vi "Populate_Do.vi"(8 "error in (no error)":errorcluster, 9 "Value":string, 10 "Lower case name":string, 11 "Build Named Build Specification in":refnum<class "Build Named Build Specification.lvclass">) -> (0 "error out":errorcluster, 1 "Success?":bool, 3 "Build Named Build Specification out":refnum<class "Build Named Build Specification.lvclass">)   [LabVIEW 2020, in "ProjectBuilder.lvlib" / "Build Named Build Specification.lvclass"]
uses:
  Build Named Build Specification.lvclass
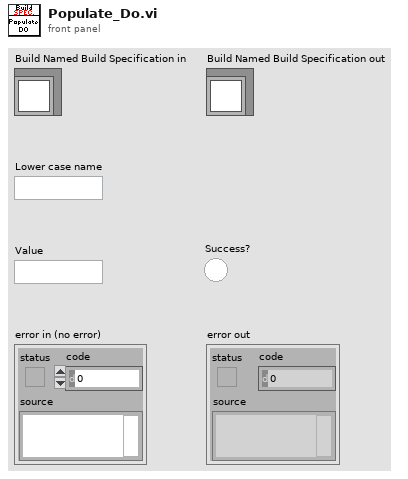
[diagram p1: front panel]
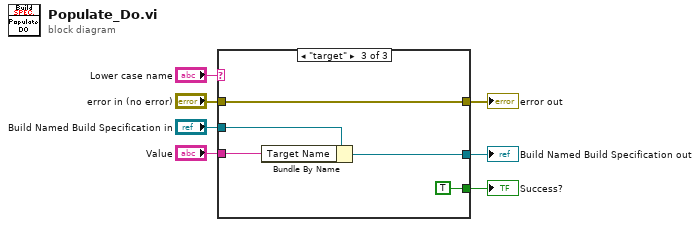
[diagram p0: block diagram]
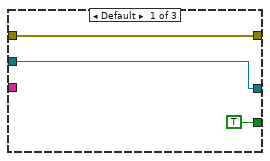
[diagram p2: hidden frame]
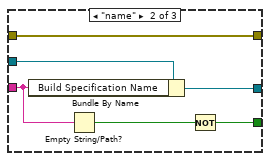
[diagram p3: hidden frame]
diagram:
  n1 = case shown="\"target\"" "Lower case name" {
    tunnel: [TRUE w12 TRUE] -> w6
    tunnel: [w9 w15 w20] -> w5
    tunnel: "Build Named Build Specification in" -> [w9 w16 w21]
    tunnel: [w8 w11 w18] -> w3
    tunnel: "error in (no error)" -> [w8 w11 w18]
    tunnel: "Value" -> [_ w14 w19]
    frame Default {
    }
    frame "name" {
      n2 = Bundle By Name(cluster=w16, "Build Specification Name"=w14) -> (w15:refnum<class "Build Named Build Specification.lvclass">)
      n3 = Empty String/Path?(string/path=w14) -> (empty?=w13:bool)
      n4 = Not(x=w13) -> (.not. x?=w12:bool)
    }
    frame "target" {
      n5 = Bundle By Name(cluster=w21, "Target Name"=w19) -> (w20:refnum<class "Build Named Build Specification.lvclass">)
    }
  }
  "error out" <- w3
  "Build Named Build Specification out" <- w5
  "Success?" <- w6
